vi "slip_filter.vi"(1 "平滑滤波输入值":dbl) -> (0 "平滑滤波输出值":dbl)   [LabVIEW 2010]
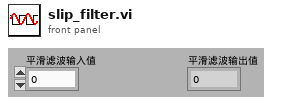
[diagram p1: front panel]
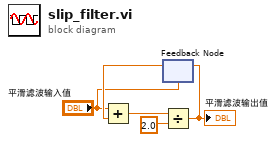
[diagram p0: block diagram]
diagram:
  n1 = feedback #1("平滑滤波输入值") -> (w2:dbl)
  n2 = Add(x="平滑滤波输入值", y=w2) -> (x+y=w5:dbl)
  n3 = Divide(x=w5, y=2.0) -> (x/y=w3:dbl)
  "平滑滤波输出值" <- w3
  n4 = feedback-in #1(w3) -> ()
